vi "Calculate Distance to Tag.vi"(6 "Enable error margin":bool=TRUE, 8 "Anchor.lvclass In":refnum<class "Anchor.lvclass">, 9 "Tag.lvclass":refnum<class "Tag.lvclass">, 10 "Error margin":dbl=3.0, 11 "DistanceLimit":dbl=90.0) -> (0 "Anchor out":refnum<class "Anchor.lvclass">, 3 "Distance":dbl)   [LabVIEW 2014, in "Anchor.lvclass"]
uses:
  Anchor.lvclass
  Tag.lvclass
panel:
  out "TagDistanceArray":T1(array[cluster])
  out "error out 3":errorcluster
  out "error out 2":errorcluster
  out "error out":errorcluster
  in  "error in (no error)":errorcluster
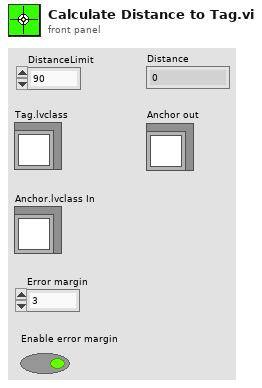
[diagram p1: front panel]
types:
  T1 = cluster{"Tag.lvclass":refnum<class "Tag.lvclass">, "Distance":dbl}[]
  T2 = cluster{"Tag out":refnum<class "Tag.lvclass">, dbl}
  T3 = cluster{"Tag out":refnum<class "Tag.lvclass">, dbl}[]
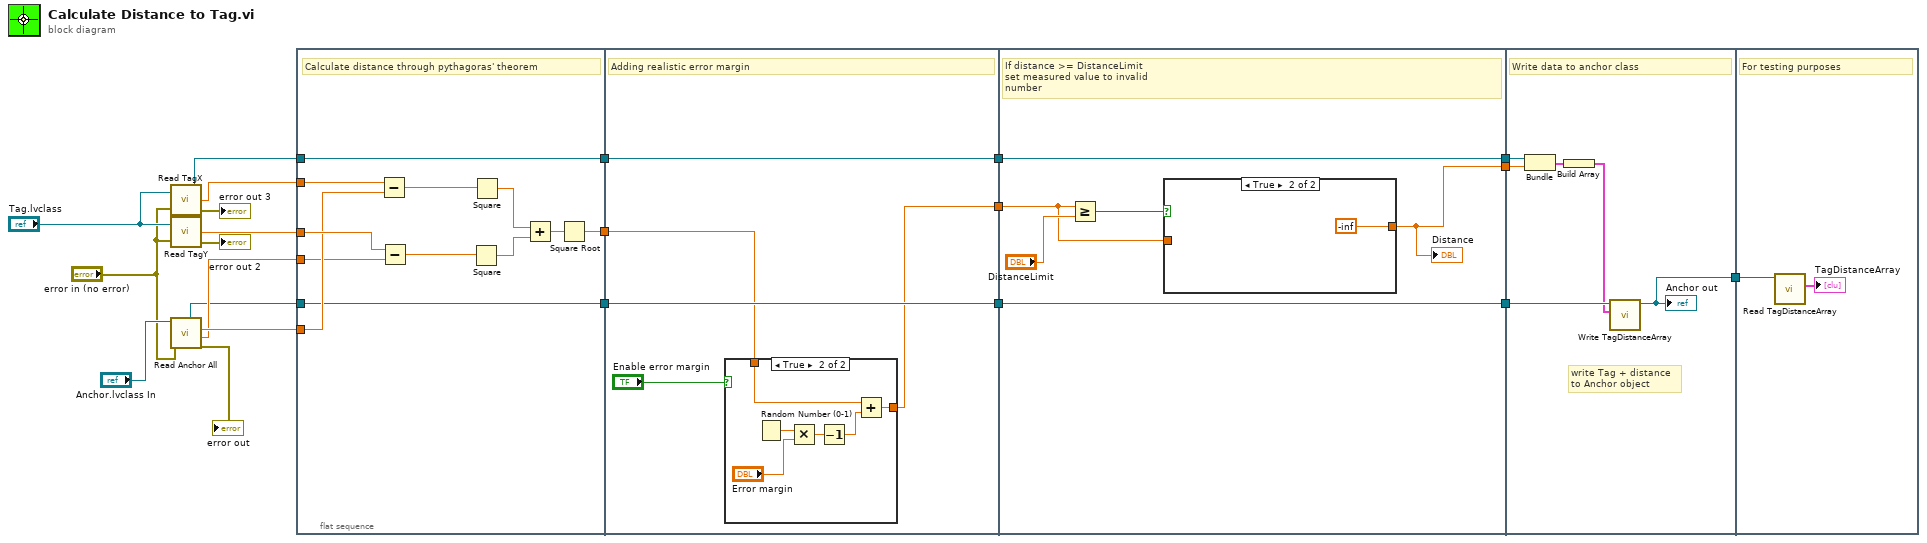
[diagram p0: block diagram]
diagram:
  n1 = call-dynamic "Read TagX.vi"("Tag in"="Tag.lvclass", "error in (no error)"="error in (no error)") -> ("Tag out"=w11:refnum<class "Tag.lvclass">, "RealTagX"=w20:dbl, "error out"=→"error out 3":errorcluster)
  n2 = call-dynamic "Read TagY.vi"("Tag in"="Tag.lvclass", "error in (no error)"="error in (no error)") -> ("RealTagY"=w19:dbl, "error out"=→"error out 2":errorcluster)  [unwired: 1 out]
  n3 = call "Read Anchor All.vi"("error in (no error)"="error in (no error)", "Anchor in"="Anchor.lvclass In") -> ("AnchorY"=w12:dbl, "AnchorX"=w13:dbl, "error out"=→"error out":errorcluster, "Anchor out"=w9:refnum<class "Anchor.lvclass">)  [unwired: 4 in, 2 out]
  n4 = flat-sequence {
    tunnel: [w29] -> w22
    tunnel: w20 -> [w28]
    tunnel: w19 -> [w27]
    tunnel: w13 -> [w26]
    tunnel: w12 -> [w25]
    tunnel: w11 -> [w24]
    tunnel: [w24] -> w10
    tunnel: w9 -> [w23]
    tunnel: [w23] -> w8
    tunnel: w22 -> [w36]
    tunnel: [w35] -> w3
    tunnel: [w39] -> w2
    tunnel: w10 -> [w39]
    tunnel: [w38] -> w1
    tunnel: w8 -> [w38]
    tunnel: w1 -> [w52]
    tunnel: [w52] -> w6
    tunnel: [w47] -> w5
    tunnel: w2 -> [w51]
    tunnel: [w51] -> w4
    tunnel: w3 -> [w48]
    tunnel: w6 -> [w60]
    tunnel: w5 -> [w58]
    tunnel: w4 -> [w59]
    tunnel: [w55] -> w7
    tunnel: w7 -> [w62]
    frame #0 {
      # "Calculate distance through pythagoras' theorem"
      n5 = Subtract(x=w28, y=w26) -> (x-y=w34:dbl)
      n6 = Subtract(x=w27, y=w25) -> (x-y=w33:dbl)
      n7 = Square(x=w33) -> (x^2=w31:dbl)
      n8 = Square(x=w34) -> (x^2=w32:dbl)
      n9 = Add(x=w32, y=w31) -> (x+y=w30:dbl)
      n10 = Square Root(x=w30) -> (sqrt(x)=w29:dbl)
    }
    frame #1 {
      # "Adding realistic error margin"
      n11 = case shown="True" "Enable error margin" {
        tunnel: w36 -> [w40 w42]
        tunnel: [w40 w41] -> w35
        frame False {
        }
        frame True {
          n12 = Random Number (0-1)() -> (number: 0 to 1=w46:dbl)
          n13 = Multiply(x=w46, y="Error margin") -> (x*y=w45:dbl)
          n14 = Decrement(x=w45) -> (x-1=w44:dbl)
          n15 = Add(x=w42, y=w44) -> (x+y=w41:dbl)
        }
      }
    }
    frame #2 {
      # "If distance >= DistanceLimit\nset measured value to invalid\nnumber"
      n16 = Greater Or Equal?(x=w48, y="DistanceLimit") -> (x >= y?=w50:bool)
      n17 = case shown="True" w50 {
        tunnel: [w53 -inf] -> w47
        tunnel: w48 -> [w53 _]
        frame False {
        }
        frame True {
        }
      }
      "Distance" <- w47
    }
    frame #3 {
      # "write Tag + distance\nto Anchor object"
      # "Write data to anchor class"
      n18 = Bundle("Tag out"=w59, w58) -> (w57:T2)  [unwired: 1 in]
      n19 = Build Array(w57) -> (w56:T3)
      n20 = call-dynamic "Write TagDistanceArray.vi"("TagDistanceArray"=w56, "Anchor in"=w60) -> ("Anchor out"=w55:refnum<class "Anchor.lvclass">)  [unwired: 8 in, 1 out]
      "Anchor out" <- w55
    }
    frame #4 {
      # "For testing purposes"
      n21 = call-dynamic "Read TagDistanceArray.vi"("Anchor in"=w62) -> ("TagDistanceArray"=→"TagDistanceArray":T1)  [unwired: 8 in, 2 out]
    }
  }
